vi "fgv_agv_speedsteer-common.vi"(7 "cmd":enum16{"init", "read", "write"}(ring), 11 "speed-steer":cluster{"speed":dbl, "steer":dbl}) -> (3 "speed-steer out":cluster{"speed":dbl, "steer":dbl})   [LabVIEW 2019]
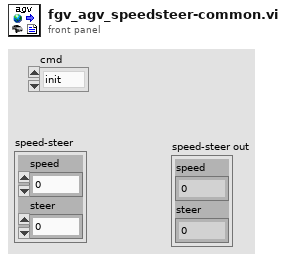
[diagram p1: front panel]
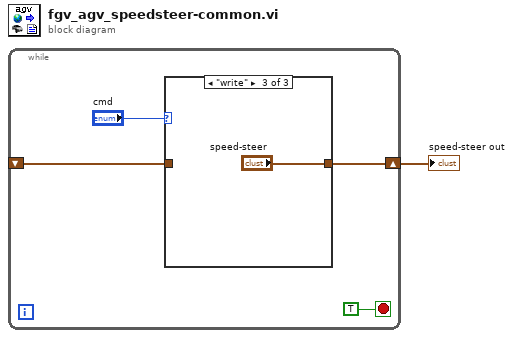
[diagram p0: block diagram]
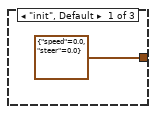
[diagram p2: hidden frame]
diagram:
  n1 = while {
    shift-right: [w3] -> w1
    shift-left: _ -> [w2]
    stop <- TRUE stop-if-true
    n2 = case shown="\"write\"" "cmd" {
      tunnel: [cluster{"speed":dbl, "steer":dbl} {"speed"=0.0, "steer"=0.0} ("t") w7 "speed-steer"] -> w3
      tunnel: w2 -> [_ w7 _]
      frame "init", Default {
      }
      frame "read" {
      }
      frame "write" {
      }
    }
  }
  "speed-steer out" <- w1
